vi "Configure.vi"(8 "error in (no error)":errorcluster, 11 "DAQMH121119OrcaFlash in":refnum<class "DAQOrcaFlash.lvclass">) -> (0 "error out":errorcluster, 2 "cancelled?":bool, 3 "DAQMH121119OrcaFlash out":refnum<class "DAQOrcaFlash.lvclass">)   [LabVIEW 2012, in "DAQOrcaFlash.lvclass"]
doc: "The configure method configures the details for the RabbitMQ connection. \n\nIn the derived class, make a call to the parent for setting these parameters."
uses:
  DAQOrcaFlash.lvclass
  trigger_source.ctl
  read out direction.ctl
  sensor_mode.ctl
  trigger_mode.ctl
  output trigger type.ctl
  connector.ctl
  output trigger period.ctl
  <vilib>/Utility/miscctls.llb/LVPointTypeDef.ctl
  DAQOrcaFlash.lvclass/DAQOrcaFlash.ctl
  <vilib>/Distrio/Murmex/Murmex/Murmex.lvclass
  output trigger source.ctl
panel:
  in  "Tab Control":T1(tab)=enum."Trigger"
  in  "Sensor mode":T2=12.0 items=["Normal"=1, "Light sheet"=12]
  in  "Read out direction":T3=1.0 items=["Top to Bottom"=1, "Bottom to Top"=2]
  in  "Output trigger period":T4=1e-05 min=5e-06 max=10 format="%#_6e"
  in  "Output trigger connector":T5
  in  "Output trigger type":T6=1.0 items=["Low"=1, "Global exposure"=2, "Programmable"=3, "Trigger ready"=4, "High"=5]
  in  "Trigger mode":T7=1.0 items=["Normal"=1, "Start"=6]
  in  "Trigger source":T8=2.0 items=["Internal"=1, "External"=2, "Software"=3]
  in  "Output trigger source":sgl(ring)=2.0 items=["READOUTEND"=2, "VSYNC"=3, "HSYNC"=4]
  in  "relay start/stop to...":i32(listbox)
  in  "button:removeRelayTarget":bool
  in  "button:addRelayTarget":bool
  in  "relay target ID":string caption="target component ID"
  in  "storage directory":path=path "R:/test_hamamatsu"
  in  "maximum window size":dbl=1024.0 caption="px"
  in  "final destination folder path (for conversion)":path
  in  "Tomo component":string
  in  "Stack component":string
  in  "auxiliary folders pahts (for conversion)":path[](array[path])
  in  "button:cancel":bool
  in  "button:ok":bool
  in  "button:configure_murmex":bool
  # "input Trigger"
  # "output trigger"
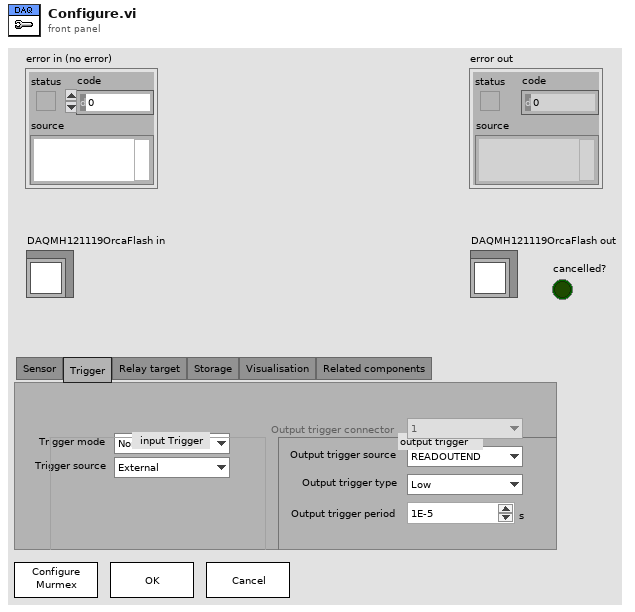
[diagram p1: front panel]
types:
  T1 = enum32{"Sensor", "Trigger", "Relay target", "Storage", "Visualisation", "Related components"}
  T2 = typedef "DAQOrcaFlash.lvclass/sensor_mode.ctl" = sgl
  T3 = typedef "DAQOrcaFlash.lvclass/read out direction.ctl" = sgl
  T4 = typedef "DAQOrcaFlash.lvclass/output trigger period.ctl" = sgl[unit]
  T5 = typedef "DAQOrcaFlash.lvclass/connector.ctl" = enum32{"1", "2", "3"}
  T6 = typedef "DAQOrcaFlash.lvclass/output trigger type.ctl" = sgl
  T7 = typedef "DAQOrcaFlash.lvclass/trigger_mode.ctl" = sgl
  T8 = typedef "DAQOrcaFlash.lvclass/trigger_source.ctl" = sgl
  T9 = enum32{"Sensor", "Trigger", "Relay target", "Storage"}
  T10 = typedef "LVPointTypeDef.ctl" = cluster{"Horizontal":i16, "Vertical":i16}
  T11 = typedef "DAQOrcaFlash.lvclass/output trigger source.ctl" = sgl
  T12 = enum8{"Enabled", "Disabled", "Disabled and Grayed Out"}
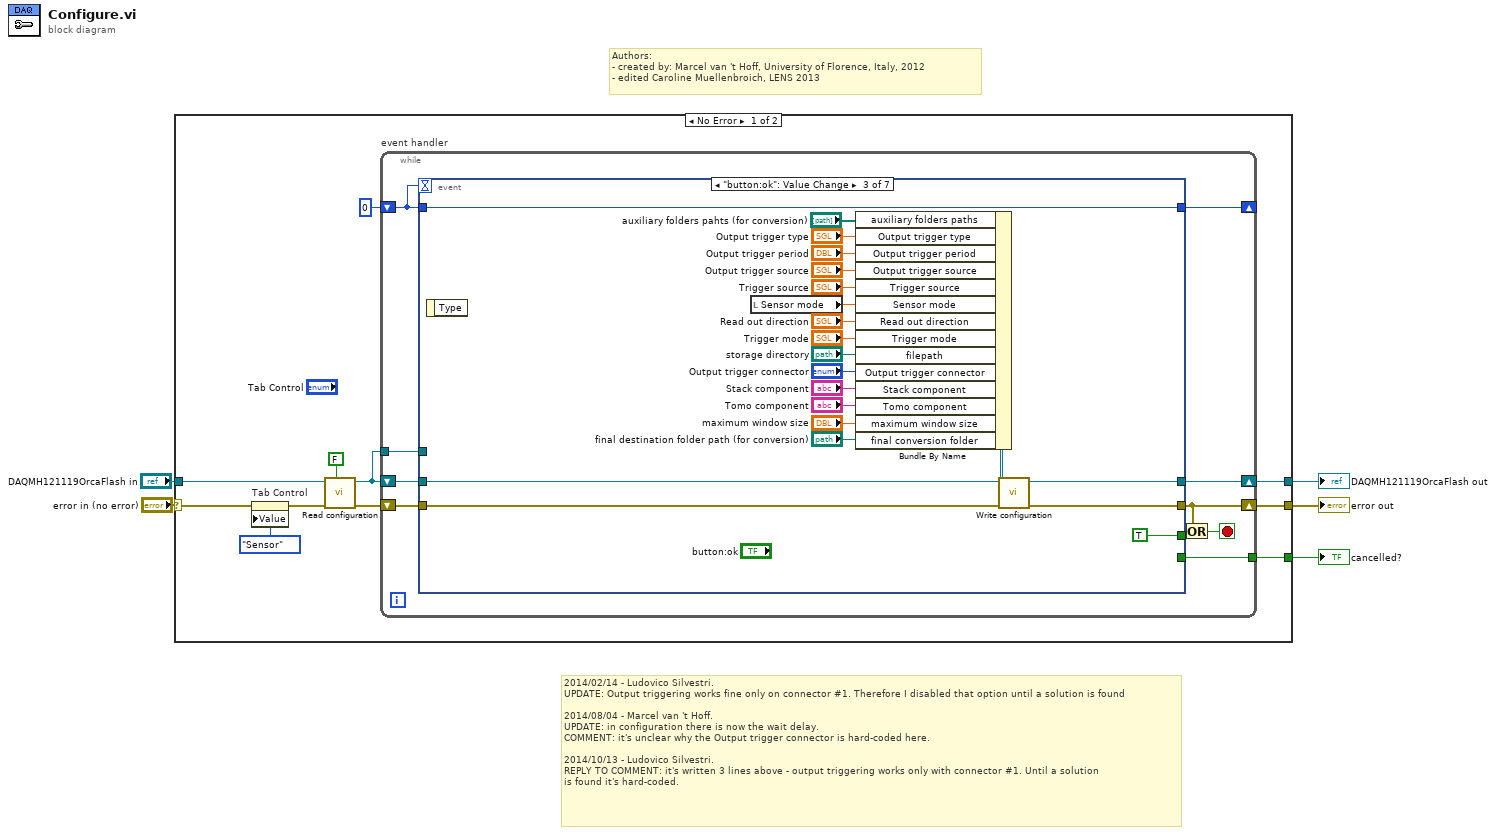
[diagram p0: block diagram]
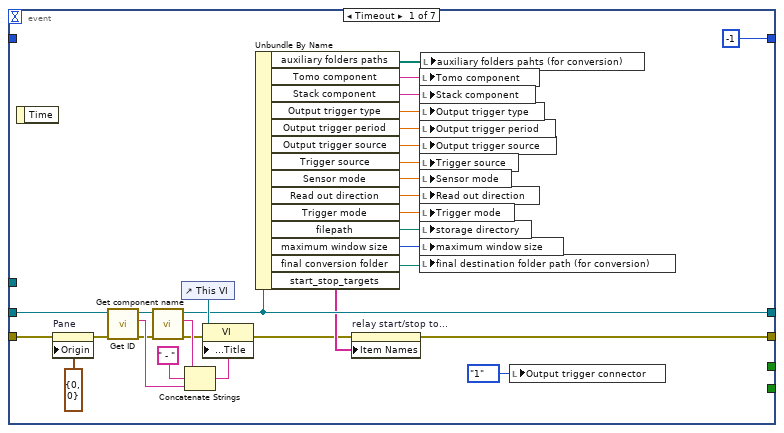
[diagram p2: hidden frame]
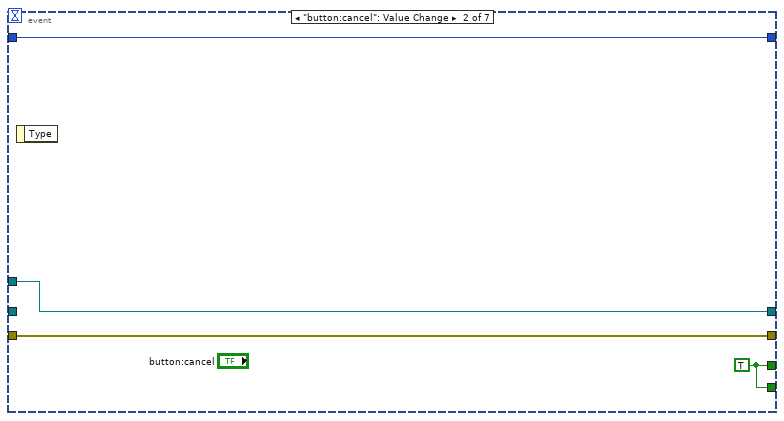
[diagram p3: hidden frame]
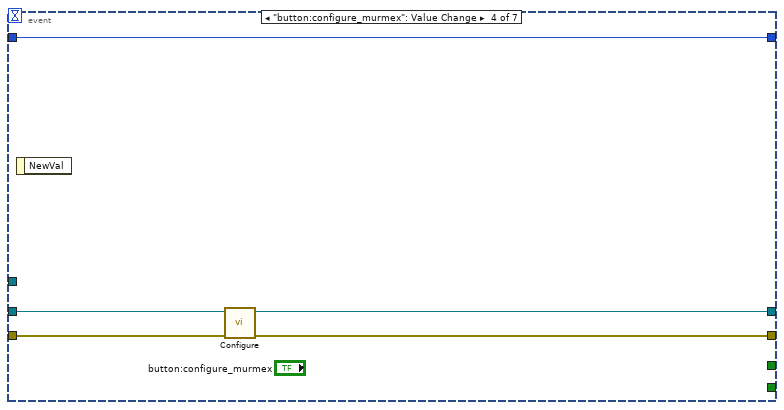
[diagram p4: hidden frame]
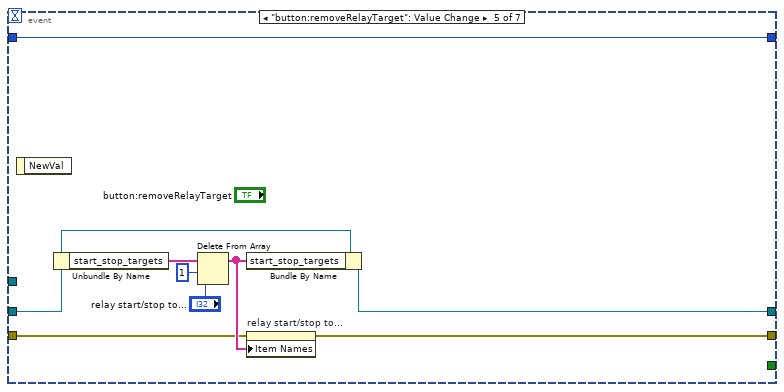
[diagram p5: hidden frame]
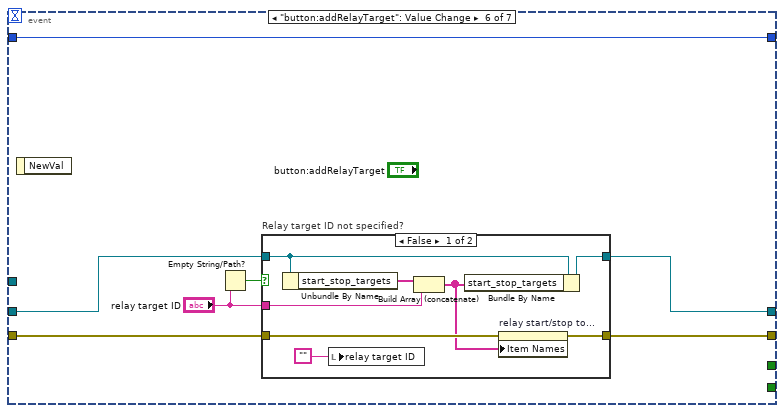
[diagram p6: hidden frame]
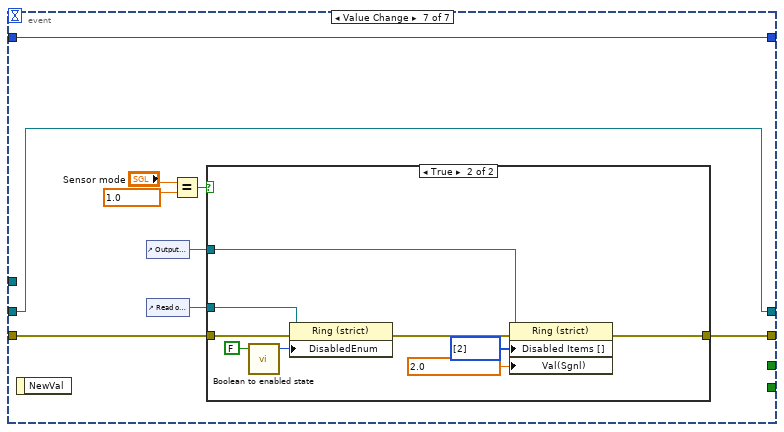
[diagram p8: hidden frame]
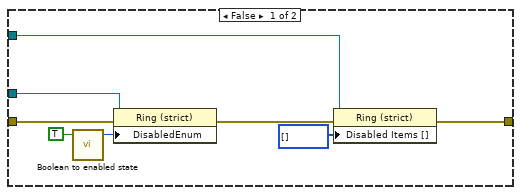
[diagram p9: hidden frame]
diagram:
  # "2014/02/14 - Ludovico Silvestri.\nUPDATE: Output triggering works fine only on connector #1. Therefore I disabled that option until a solution is found\n\n2014/08/04 - Marcel van 't Hoff.\nUPDATE: in configuration there is now the wait delay.\nCOMMENT: it's unclear why the Output trigger connector is hard-coded here.\n\n2014/10/13 - Ludovico Silvestri.\nREPLY TO COMMENT: it's written 3 lines above - output triggering works only with connector #1. Until a solution\nis found it's hard-coded."
  # "Authors: \n- created by: Marcel van 't Hoff, University of Florence, Italy, 2012\n- edited Caroline Muellenbroich, LENS 2013"
  n1 = case shown="No Error" "error in (no error)" {
    selector: "error in (no error)" -> [w7 w140]
    tunnel: [w16 w140] -> w5
    tunnel: [w15 w141] -> w1
    tunnel: [w13 _] -> w4
    tunnel: "DAQMH121119OrcaFlash in" -> [w10 w141]
    frame No Error {
      n2 = property on="Tab Control" class="TabCtl (strict)"(error in=w7, "Value"=T9."Sensor" ("Tab Control")) -> (error out=w6:errorcluster)  [unwired: 1 in, 1 out]
      n3 = call-dynamic "Read configuration.vi"("force loading?"=FALSE, "error in (no error)"=w6, "DAQMH121119OrcaFlash in"=w10) -> ("error out"=w11:errorcluster, "DAQMH121119OrcaFlash out"=w9:refnum<class "DAQOrcaFlash.lvclass">)  [unwired: 7 in]
      n4 = while "event handler" {
        shift-right: [w23] -> w16
        shift-left: w11 -> [w25]
        shift-right: [w26] -> w15
        shift-left: w9 -> [w24]
        shift-right: [w21] -> _
        shift-left: 0 -> [w20]
        tunnel: [w18] -> w13
        tunnel: w9 -> [w17]
        stop <- w22 stop-if-true
        n5 = event shown="[2] \"button:ok\": Value Change" {
          selector: _ -> [_ _ _ _ _ _ _]
          dyn-events: _ -> [_ _ _ _ _ _ _]
          timeout: w20 -> [_ _ _ _ _ _ _]
          tunnel: [w33 w61 w79 w87 w89 w98 w115] -> w23
          tunnel: [w36 w58 w78 w86 w93 w100 w114] -> w26
          tunnel: w25 -> [w54 w61 w82 w85 w90 w99 w118]
          tunnel: w24 -> [w57 _ w77 w84 w94 w101 w114]
          tunnel: [-1 w60 w81 w83 w88 w97 w122] -> w21
          tunnel: w20 -> [_ w60 w81 w83 w88 w97 w122]
          tunnel: [_ w59 TRUE _ _ _ _] -> w19
          tunnel: [_ w59 _ _ _ _ _] -> w18
          tunnel: w17 -> [_ w58 _ _ _ _ _]
          event Timeout {
            n6 = event-data() -> ()  [unwired: 1 in, 1 out]
            n7 = property on="Pane" class="Pane"(error in=w54, "Origin"=T10 {"Horizontal"=0, "Vertical"=0}) -> (error out=w49:errorcluster)  [unwired: 1 in, 1 out]
            n8 = call <vilib>:"Get ID.vi"("error in (no error)"=w49, "Murmex in"=w57) -> ("error out"=w48:errorcluster, "component id"=w51:string, "Murmex out"=w53:refnum<class "DAQOrcaFlash.lvclass">)  [unwired: 7 in]
            n9 = call <vilib>:"Get component name.vi"("error in (no error)"=w48, "Murmex in"=w53) -> ("error out"=w37:errorcluster, "component name"=w52:string, "Murmex out"=w36:refnum<class "DAQOrcaFlash.lvclass">)  [unwired: 7 in]
            n10 = control-ref of="This VI"() -> (w38:refnum<vi>)
            n11 = Concatenate Strings(w52, " - " ("string"), w51) -> (w39:string)
            n12 = property class="VI"(reference=w38, error in=w37, "Front Panel.Title"=w39) -> (error out=w34:errorcluster)  [unwired: 1 out]
            n13 = Unbundle By Name(w36) -> ("auxiliary folders paths"=w29:path[], "Tomo component"=w30:string, "Stack component"=w31:string, "Output trigger type"=w40:T6, "Output trigger period"=w41:sgl[unit], "Output trigger source"=w42:T11, "Trigger source"=w46:T8, "Sensor mode"=w45:T2, "Read out direction"=w44:T3, "Trigger mode"=w43:T7, "filepath"=w47:path, "maximum window size"=w28:i32, "final conversion folder"=w27:path, "start_stop_targets"=w35:string[])
            n14 = property on="relay start/stop to..." class="LstBox (strict)"(error in=w34, "Item Names"=w35) -> (error out=w33:errorcluster)  [unwired: 1 in, 1 out]
            n15 = local write "Tomo component"(w30) -> ()
            n16 = local write "Stack component"(w31) -> ()
            n17 = local write "Output trigger type"(w40) -> ()
            n18 = local write "Output trigger period"(w41) -> ()
            n19 = local write "Output trigger source"(w42) -> ()
            n20 = local write "Trigger source"(w46) -> ()
            n21 = local write "Sensor mode"(w45) -> ()
            n22 = local write "Read out direction"(w44) -> ()
            n23 = local write "Trigger mode"(w43) -> ()
            n24 = local write "storage directory"(w47) -> ()
            n25 = local write "maximum window size"(w28) -> ()
            n26 = local write "final destination folder path (for conversion)"(w27) -> ()
            n27 = local write "auxiliary folders pahts (for conversion)"(w29) -> ()
            n28 = local write "Output trigger connector"(connector."1" ("configuration.Output trigger connector")) -> ()
          }
          event "button:cancel": Value Change {
            w59 = TRUE
            n29 = event-data() -> ()  [unwired: 1 in, 1 out]
          }
          event "button:ok": Value Change {
            n30 = event-data() -> ()  [unwired: 1 in, 1 out]
            n31 = local read "Sensor mode"() -> (w68:T2)
            n32 = Bundle By Name(cluster=w77, "auxiliary folders paths"="auxiliary folders pahts (for conversion)", "Output trigger type"="Output trigger type", "Output trigger period"="Output trigger period", "Output trigger source"="Output trigger source", "Trigger source"="Trigger source", "Sensor mode"=w68, "Read out direction"="Read out direction", "Trigger mode"="Trigger mode", "filepath"="storage directory", "Output trigger connector"="Output trigger connector", "Stack component"="Stack component", "Tomo component"="Tomo component", "maximum window size"="maximum window size", "final conversion folder"="final destination folder path (for conversion)") -> (w76:refnum<class "DAQOrcaFlash.lvclass">)
            n33 = call-dynamic "Write configuration.vi"("error in (no error)"=w82, "DAQMH121119OrcaFlash in"=w76) -> ("error out"=w79:errorcluster, "DAQMH121119OrcaFlash out"=w78:refnum<class "DAQOrcaFlash.lvclass">)  [unwired: 8 in]
          }
          event "button:configure_murmex": Value Change {
            n34 = event-data() -> ()  [unwired: 1 in, 1 out]
            n35 = call-parent "Configure.vi"("error in (no error)"=w85, "Murmex in"=w84) -> ("error out"=w87:errorcluster, "Murmex out"=w86:refnum<class "DAQOrcaFlash.lvclass">)  [unwired: 7 in, 1 out]
          }
          event "button:removeRelayTarget": Value Change {
            n36 = event-data() -> ()  [unwired: 1 in, 1 out]
            n37 = Unbundle By Name(w94) -> ("start_stop_targets"=w96:string[])
            n38 = Delete From Array(array=w96, length=1, index="relay start/stop to...") -> (array with subset deleted=w91:string[])  [unwired: 1 out]
            n39 = Bundle By Name(cluster=w94, "start_stop_targets"=w91) -> (w93:refnum<class "DAQOrcaFlash.lvclass">)
            n40 = property on="relay start/stop to..." class="LstBox (strict)"(error in=w90, "Item Names"=w91) -> (error out=w89:errorcluster)  [unwired: 1 in, 1 out]
          }
          event "button:addRelayTarget": Value Change {
            n41 = event-data() -> ()  [unwired: 1 in, 1 out]
            n42 = Empty String/Path?(string/path="relay target ID") -> (empty?=w103:bool)
            n43 = case "Relay target ID not specified?" shown="False" w103 {
              tunnel: w101 -> [w110 w113]
              tunnel: [w109 w113] -> w100
              tunnel: "relay target ID" -> [w108 _]
              tunnel: w99 -> [w106 w112]
              tunnel: [w105 w112] -> w98
              frame False {
                n44 = Unbundle By Name(w110) -> ("start_stop_targets"=w111:string[])
                n45 = local write "relay target ID"("") -> ()
                n46 = Build Array (concatenate)(w111, w108) -> (w104:string[])
                n47 = Bundle By Name(cluster=w110, "start_stop_targets"=w104) -> (w109:refnum<class "DAQOrcaFlash.lvclass">)
                n48 = property on="relay start/stop to..." class="LstBox (strict)"(error in=w106, "Item Names"=w104) -> (error out=w105:errorcluster)  [unwired: 1 in, 1 out]
              }
              frame True {
              }
            }
          }
          event Value Change {
            w120 = T2 1.0 items=["Normal"=1.0, "Light sheet"=12.0] ("y")
            n49 = event-data() -> ()  [unwired: 1 in, 1 out]
            n50 = control-ref of="Output trigger source"() -> (w116:refnum<vi>)
            n51 = control-ref of="Read out direction"() -> (w117:refnum<vi>)
            n52 = Equal?(x="Sensor mode", y=w120) -> (x = y?=w119:bool)
            n53 = case shown="True" w119 {
              tunnel: w118 -> [w127 w138]
              tunnel: w117 -> [w126 w139]
              tunnel: w116 -> [w125 w135]
              tunnel: [w123 w133] -> w115
              frame False {
                n54 = call <vilib>:"Boolean to enabled state.vi"("boolean in"=TRUE) -> ("enabled status out"=w130:T12)  [unwired: 4 in]
                n55 = property class="Ring (strict)"(reference=w126, error in=w127, "DisabledEnum"=w130) -> (error out=w128:errorcluster)  [unwired: 1 out]
                n56 = property class="Ring (strict)"(reference=w125, error in=w128, "Disabled Items []"=i32[] []) -> (error out=w123:errorcluster)  [unwired: 1 out]
              }
              frame True {
                w131 = T11 2.0 items=["READOUTEND"=2.0, "VSYNC"=3.0, "HSYNC"=4.0] ("Value (Signaling)")
                n57 = call <vilib>:"Boolean to enabled state.vi"("boolean in"=FALSE) -> ("enabled status out"=w137:T12)  [unwired: 4 in]
                n58 = property class="Ring (strict)"(reference=w139, error in=w138, "DisabledEnum"=w137) -> (error out=w134:errorcluster)  [unwired: 1 out]
                n59 = property class="Ring (strict)"(reference=w135, error in=w134, "Disabled Items []"=i32[] [2], "Val(Sgnl)"=w131) -> (error out=w133:errorcluster)  [unwired: 1 out]
              }
            }
          }
        }
        n60 = Or(x=w23, y=w19) -> (x .or. y?=w22:bool)
      }
    }
    frame Error {
    }
  }
  "error out" <- w5
  "DAQMH121119OrcaFlash out" <- w1
  "cancelled?" <- w4
